vi "Compile CHM.vi"(8 "error in (no error)":errorcluster, 11 "CHM Generator in":refnum<class "CHM Generator.lvclass">) -> (0 "error out":errorcluster, 2 "standard output":string, 3 "CHM Generator out":refnum<class "CHM Generator.lvclass">)   [LabVIEW 2015, in "CHM Generator.lvclass"]
uses:
  CHM Generator.lvclass
  <vilib>/Utility/sysdir.llb/System Directory Type.ctl
  CHM Generator.lvclass/CHM Generator.ctl
  Keyed Value Tree/Keyed Value Tree.lvclass
panel:
  out "return code":i32
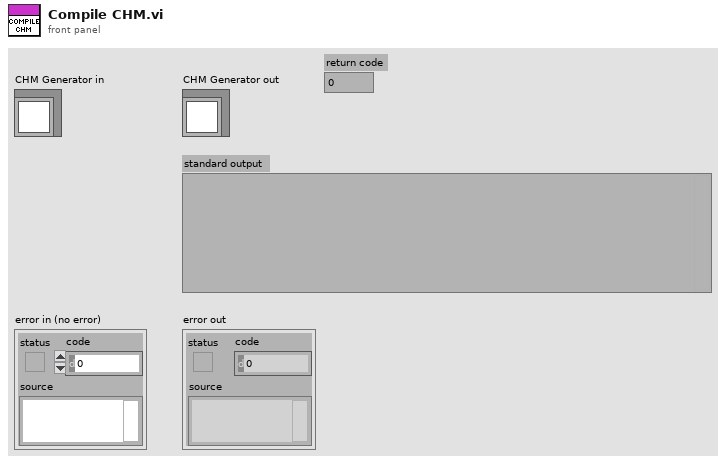
[diagram p1: front panel]
types:
  T1 = typedef "System Directory Type.ctl" = i32
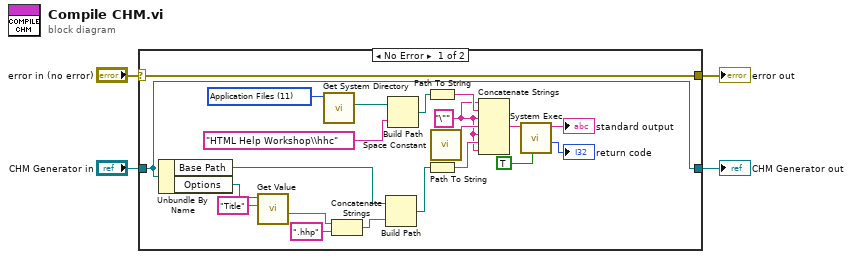
[diagram p0: block diagram]
diagram:
  n1 = case shown="No Error" "error in (no error)" {
    selector: "error in (no error)" -> [w25 w27]
    tunnel: [w25 w27] -> w3
    tunnel: [w24 w26] -> w1
    tunnel: "CHM Generator in" -> [w24 w26]
    frame No Error {
      w13 = "\"" ("string")
      w18 = T1 11 items=["User Home"=0, "User Desktop"=1, "User Documents"=2, "User Application Data"=3, "User Preferences"=4, "User Temporary"=5, "Public Documents"=6, "Public Application Data"=7, "Public Preferences"=8, "Public Cache"=13, "System Core Libraries"=9, "System Installed Libraries"=10, "Application Files"=11, "Boot Volume Root"=12] ("system directory type")
      n2 = Unbundle By Name(w24) -> ("Base Path"=w7:path, "Options"=w12:refnum<class "Keyed Value Tree.lvclass">)
      n3 = call-dynamic "Get Value.vi"("name"="Title", "Keyed Value Tree in"=w12) -> ("value"=w10:string)  [unwired: 6 in, 3 out]
      n4 = call <vilib>:"Get System Directory.vi"("system directory type"=w18) -> ("system directory"=w16:path)  [unwired: 10 in]
      n5 = Concatenate Strings(w10, ".hhp" ("string")) -> (w8:string)
      n6 = Build Path(base path=w7, name or relative path=w8) -> (appended path=w6:path)
      n7 = Build Path(base path=w16, name or relative path="HTML Help Workshop\\hhc") -> (appended path=w14:path)
      n8 = Path To String(path=w14) -> (string=w17:string)
      n9 = Path To String(path=w6) -> (string=w22:string)
      n10 = call <vilib>:"Space Constant.vi"() -> ("String"=w21:string)
      n11 = Concatenate Strings(w13, w17, w13, w21, w13, w22, w13) -> (w23:string)
      n12 = call <vilib>:"System Exec.vi"("run minimized? (F)"=TRUE, "command line"=w23) -> ("return code"=→"return code":i32, "standard output"=→"standard output":string)  [unwired: 6 in, 2 out]
    }
    frame Error {
    }
  }
  "error out" <- w3
  "CHM Generator out" <- w1
